vi "2.vi"() -> ()   [LabVIEW 2013]
uses:
  <vilib>/Math Plots/3D Math Plots/3D Surface/3D Surface XCtrl/3D Surface.xctl
  <vilib>/Math Plots/3D Math Plots/3D Surface/3D Surface Datatype/Public/Plot Helper (Vector).vi
  <vilib>/express/express arith-compare/Formula/XNode/ExpressFormulaBlockNode.xnode
  <vilib>/Math Plots/3D Math Plots/3D Surface/3D Surface Datatype/3D Surface Datatype.lvclass
panel:
  in  "Y = 0 ?":bool
  out "3D Surface":refnum<class "3D Plot Datatype.lvclass">[](xcontrol)
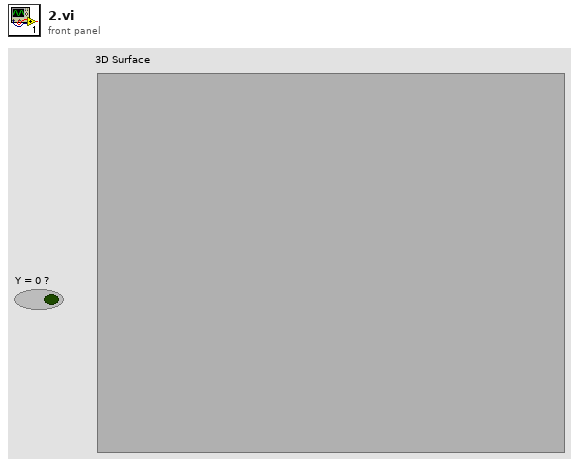
[diagram p1: front panel]
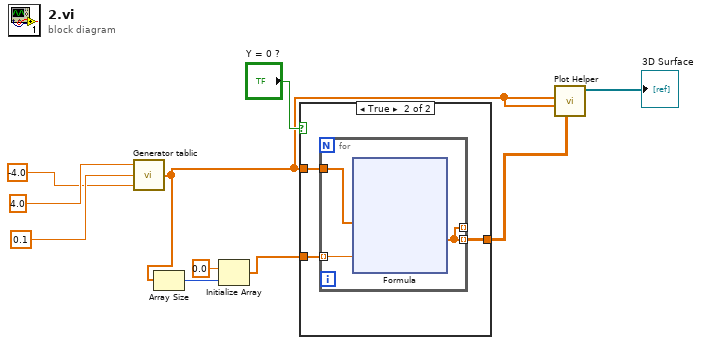
[diagram p0: block diagram]
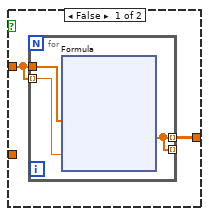
[diagram p2: hidden frame]
diagram:
  n1 = call "Generator tablic.vi"("Start"=-4.0 ("End"), "Krok"=0.1, "End"=4.0 ("Start")) -> ("Array"=w3:dbl[])
  n2 = Array Size(array=w3) -> (size(s)=w4:i32)
  n3 = Initialize Array(0.0 ("element"), w4) -> (w1:dbl[])
  n4 = case shown="True" "Y = 0 ?" {
    tunnel: w3 -> [w11 w31]
    tunnel: [w12 w29] -> w9
    tunnel: w1 -> [_ w30]
    frame False {
      n5 = for {
        tunnel: w11 -> [w15]
        tunnel: w11 -> [w14] mode=indexing
        tunnel: [w13] -> _ mode=indexing
        tunnel: [w13] -> w12 mode=indexing
        n6 = xnode "Formula"("x"=w15, "y"=w14) -> ("Result"=w13:dbl[])  [unwired: 1 in, 1 out]
      }
    }
    frame True {
      n7 = for {
        tunnel: w31 -> [w34]
        tunnel: w30 -> [w33] mode=indexing
        tunnel: [w32] -> w29 mode=indexing
        tunnel: [w32] -> _ mode=indexing
        n8 = xnode "Formula"("x"=w34, "y"=w33) -> ("Result"=w32:dbl[])  [unwired: 1 in, 1 out]
      }
    }
  }
  n9 = call-poly <vilib>:"Plot Helper.vi"("z matrix"=w9, "y vector"=w3, "x vector"=w3) -> ("3D Plot lvclass Array out"=→"3D Surface":refnum<class "3D Plot Datatype.lvclass">[])  [unwired: 3 in, 5 out]
